vi "About Button.vi"(11 "Called?":bool) -> ()   [LabVIEW 2023]
uses:
  Controls/DisplayQCommand.ctl
  Controls/DisplayMessage.ctl
panel:
  in  "About":bool
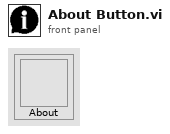
[diagram p1: front panel]
types:
  T1 = enum8{"Enabled", "Disabled", "Disabled and Grayed Out"}
  T2 = typedef "DisplayMessage.ctl" = enum16{"No Message - Ignore", "Display Message", "Set Tab", "Set Status", "Add Error Message", "Clear Error History", "Generate Error", "Set Idling Display", "Set Running Display", "Set Subpanel Output", "Stop"}
  T3 = typedef "DisplayQCommand.ctl" = enum16{"No Command - Error", "Initialise", "Get Q Reference", "Add Item to Bottom", "Add Item to Top", "Flush Q", "Dequeue", "Peek Next Element", "Close"}
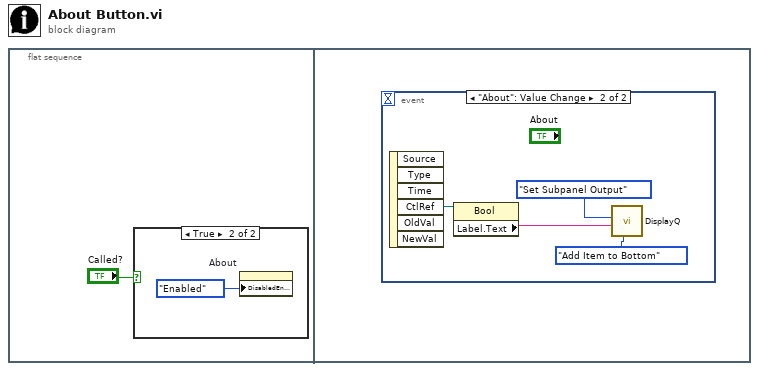
[diagram p0: block diagram]
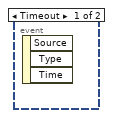
[diagram p3: hidden frame]
diagram:
  n1 = flat-sequence {
    frame #0 {
      n2 = case shown="True" "Called?" {
        frame False {
        }
        frame True {
          n3 = property on="About" class="Bool"("DisabledEnum"=T1."Enabled" ("Disabled")) -> ()  [unwired: 2 in, 2 out]
        }
      }
    }
    frame #1 {
      n4 = event shown="[1] \"About\": Value Change" {
        selector: _ -> [_ _]
        dyn-events: _ -> [_ _]
        timeout: _ -> [_ _]
        event Timeout {
          n5 = event-data() -> ()  [unwired: 1 in, 3 out]
        }
        event "About": Value Change {
          n6 = event-data() -> ("CtlRef"=w4:refnum<vi>)  [unwired: 1 in, 5 out]
          n7 = property class="Bool"(reference=w4) -> ("Label.Text"=w3:string)  [unwired: 1 in, 2 out]
          n8 = call "DisplayQ.vi"("command"=DisplayQCommand."Add Item to Bottom", "DataIn"=w3, "DisplayMessage"=DisplayMessage."Set Subpanel Output") -> ()  [unwired: 2 in, 4 out]
        }
      }
    }
  }
